vi "Get Image.vi"(8 "error in (no error)":errorcluster, 11 "Dell Webcam in":refnum<class "Webcam.lvclass">) -> (0 "error out":errorcluster, 2 "Image Reference":T1, 3 "Dell Webcam out":refnum<class "Webcam.lvclass">)   [LabVIEW 2019, in "Webcam.lvclass"]
uses:
  Webcam.lvclass
  <vilib>/vision/Image Controls.llb/IMAQ Image.ctl
  Webcam.lvclass/Webcam.ctl
  <vilib>/vision/driver/NI_Vision_Acquisition_Software.lvlib
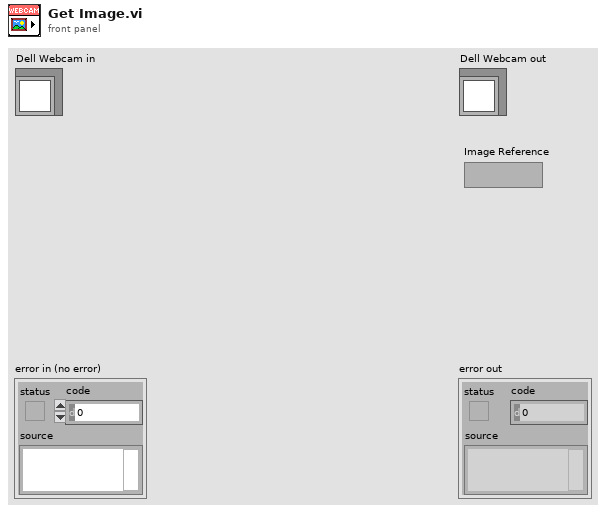
[diagram p1: front panel]
types:
  T1 = typedef "IMAQ Image.ctl" = refnum<image>
  T2 = typedef "IMAQdx.ctl" = refnum<k21>
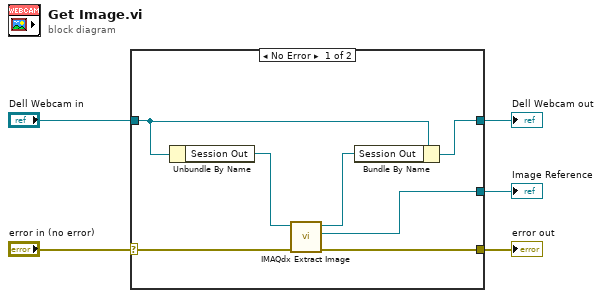
[diagram p0: block diagram]
diagram:
  n1 = case shown="No Error" "error in (no error)" {
    selector: "error in (no error)" -> [w12 w13]
    tunnel: [w11 w13] -> w4
    tunnel: "Dell Webcam in" -> [w10 w14]
    tunnel: [w7 w14] -> w2
    tunnel: [w6 _] -> w1
    frame No Error {
      n2 = Unbundle By Name(w10) -> ("Session Out"=w9:T2)
      n3 = call <vilib>:"IMAQdx Extract Image.vi"("error in"=w12, "Session In"=w9) -> ("error out"=w11:errorcluster, "Image Out"=w6:T1, "Session Out"=w8:T2)  [unwired: 6 in, 1 out]
      n4 = Bundle By Name(cluster=w10, "Session Out"=w8) -> (w7:refnum<class "Webcam.lvclass">)
    }
    frame Error {
    }
  }
  "error out" <- w4
  "Dell Webcam out" <- w2
  "Image Reference" <- w1
